vi "G4BaseTemplate_Simple_6x8x6_NoneModifing.vi"(0 "reference in":refnum<class "G4BaseTemplate_Simple_6x8x6.lvclass">, 5 "error in (no error)":errorcluster) -> (14 "reference out":refnum<class "G4BaseTemplate_Simple_6x8x6.lvclass">, 19 "error out":errorcluster)   [LabVIEW 2010]
uses:
  G4BaseTemplate_Simple_6x8x6.lvclass
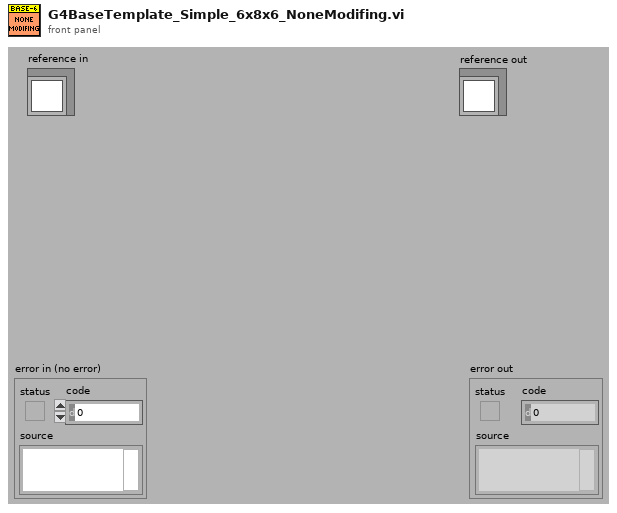
[diagram p1: front panel]
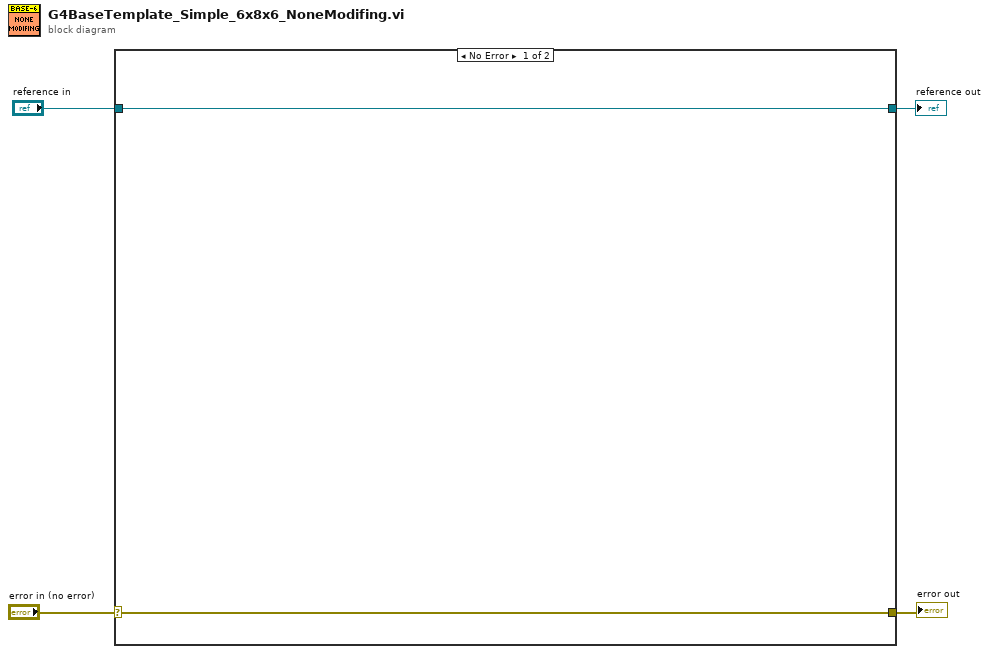
[diagram p0: block diagram]
diagram:
  n1 = case shown="No Error" "error in (no error)" {
    selector: "error in (no error)" -> [w5 w8]
    tunnel: [w5 w8] -> w3
    tunnel: [w6 w7] -> w1
    tunnel: "reference in" -> [w6 w7]
    frame No Error {
    }
    frame Error {
    }
  }
  "error out" <- w3
  "reference out" <- w1
